vi "Driver Retrieve Record.vi"(8 "error in (no error)":errorcluster, 11 "Statement Refnum":T2) -> (0 "error out":errorcluster, 2 "Driver Record":T1, 3 "Statement Refnum":T2)   [LabVIEW 2011]
uses:
  Summitek EXT/ODBC/SQL Controls/Statement Refnum.ctl
  Driver Record.ctl
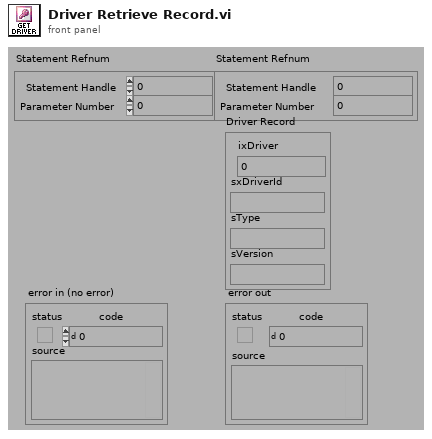
[diagram p1: front panel]
types:
  T1 = typedef "Driver Record.ctl" = cluster{"ixDriver":i32, "sxDriverId":string, "sType":string, "sVersion":string}
  T2 = typedef "Statement Refnum.ctl" = cluster{"Statement Handle":i32, "Parameter Number":u16}
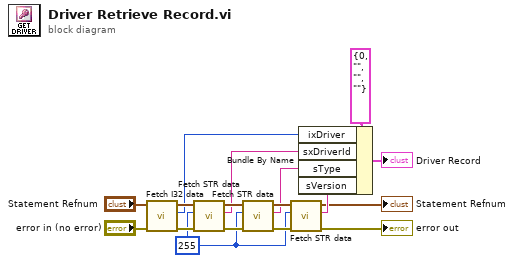
[diagram p0: block diagram]
diagram:
  w9 = 255 ("Buffer Size")
  n1 = call "Fetch I32 data.vi"("error in (no error)"="error in (no error)", "Statement Refnum"="Statement Refnum") -> ("error out"=w14:errorcluster, "Data"=w12:i32, "Statement Refnum"=w13:T2)  [unwired: 3 out]
  n2 = call "Fetch STR data.vi"("error in (no error)"=w14, "Buffer Size"=w9, "Statement Refnum"=w13) -> ("error out"=w16:errorcluster, "Data"=w5:string, "Statement Refnum"=w15:T2)  [unwired: 2 out]
  n3 = call "Fetch STR data.vi"("error in (no error)"=w16, "Buffer Size"=w9, "Statement Refnum"=w15) -> ("error out"=w11:errorcluster, "Data"=w4:string, "Statement Refnum"=w10:T2)  [unwired: 2 out]
  n4 = call "Fetch STR data.vi"("error in (no error)"=w11, "Buffer Size"=w9, "Statement Refnum"=w10) -> ("error out"=→"error out":errorcluster, "Data"=w6:string, "Statement Refnum"=→"Statement Refnum":T2)  [unwired: 2 out]
  n5 = Bundle By Name(cluster=T1 {"ixDriver"=0, "sxDriverId"="", "sType"="", "sVersion"=""} ("Station Information"), "ixDriver"=w12, "sxDriverId"=w5, "sType"=w4, "sVersion"=w6) -> (→"Driver Record":T1)
